vi "Find some Public API VI.vi"(7 "Theme":bool=TRUE, 8 "Public Api file index":i32, 9 "Library in":refnum<vi>, 10 "Target":refnum<vi>, 11 "App Ref":refnum<vi>) -> ()   [LabVIEW 2019, in "Panther Dashboard.lvlib"]
uses:
  Panther Dashboard.lvlib
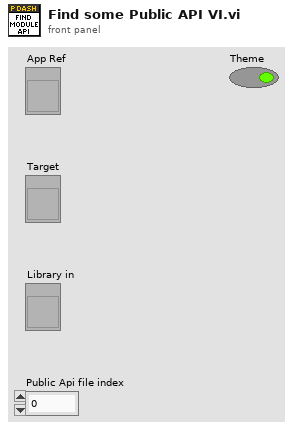
[diagram p1: front panel]
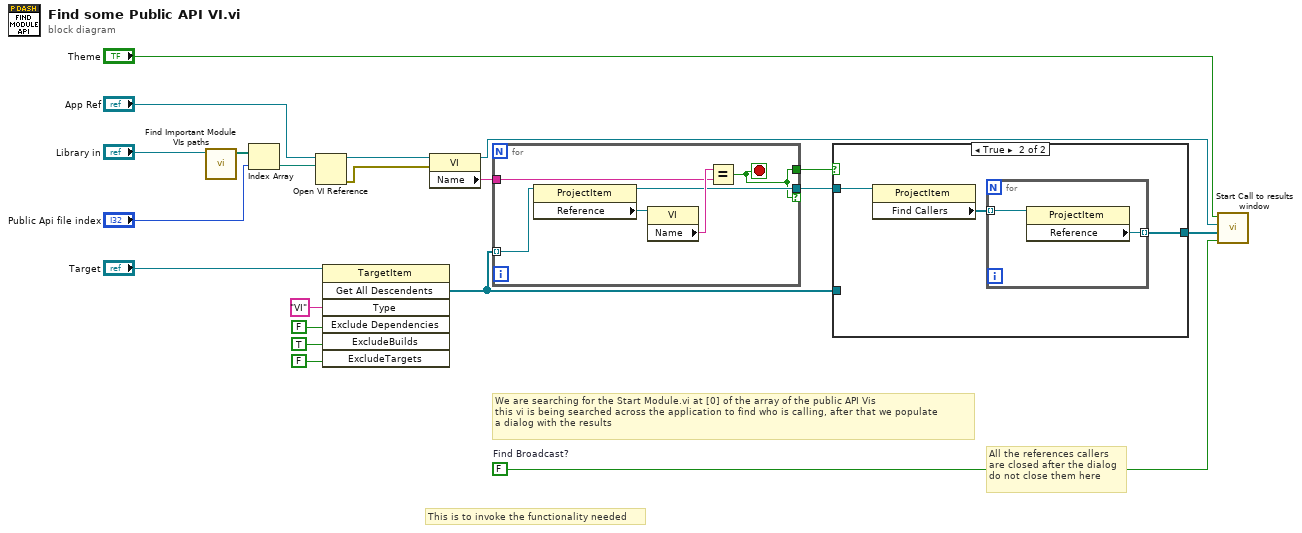
[diagram p0: block diagram]
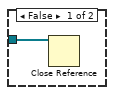
[diagram p2: hidden frame]
diagram:
  w4 = FALSE  # Find Broadcast?
  # "All the references callers\nare closed after the dialog\ndo not close them here"
  # "This is to invoke the functionality needed"
  # "We are searching for the Start Module.vi at [0] of the array of the public API Vis\nthis vi is being searched across the application to find who is calling, after that we populate\na dialog with the results"
  n1 = call "Find Important Module VIs paths.vi"("Library in"="Library in") -> ("Public API VIs Paths"=w18:path[])  [unwired: 10 in]
  n2 = Index Array(array=w18, index="Public Api file index") -> (element=w17:path)
  n3 = Open VI Reference(application reference (local)="App Ref", vi path=w17) -> (vi reference=w5:refnum<vi>, error out=w20:errorcluster)  [unwired: 4 in]
  n4 = invoke class="TargetItem" method="Get All Descendents"(reference="Target", "Type"="VI", "Exclude Dependencies"=FALSE ("ExcludeDependencies"), "ExcludeBuilds"=TRUE, "ExcludeTargets"=FALSE) -> ("All Descendents"=w6:refnum<vi>[])  [unwired: 2 in, 6 out]
  n5 = property class="VI"(reference=w5, error in=w20) -> (reference out=w1:refnum<vi>, "Name"=w13:string)  [unwired: 1 out]
  n6 = for {
    tunnel: w6 -> [w26] mode=indexing
    tunnel: w13 -> [w23]
    tunnel: [w22] -> w11 if=w21
    tunnel: [w21] -> w12
    stop <- w21 stop-if-true
    n7 = property class="ProjectItem"(reference=w26) -> (reference out=w22:refnum<vi>, "Reference"=w25:refnum<vi>)  [unwired: 1 in, 1 out]
    n8 = property class="VI"(reference=w25) -> ("Name"=w24:string)  [unwired: 1 in, 2 out]
    n9 = Equal?(x=w24, y=w23) -> (x = y?=w21:bool)
  }
  n10 = case shown="True" w12 {
    tunnel: w11 -> [_ w30]
    tunnel: w6 -> [w27 _]
    tunnel: [_ w28] -> w3
    frame False {
      n11 = Close Reference(reference=w27) -> ()  [unwired: 1 in, 1 out]
    }
    frame True {
      n12 = property class="ProjectItem"(reference=w30) -> ("Find Callers"=w29:refnum<vi>[])  [unwired: 1 in, 2 out]
      n13 = for {
        tunnel: w29 -> [w32] mode=indexing
        tunnel: [w31] -> w28 mode=indexing
        n14 = property class="ProjectItem"(reference=w32) -> ("Reference"=w31:refnum<vi>)  [unwired: 1 in, 2 out]
      }
    }
  }
  n15 = call "Start Call to results window.vi"("Find Broadcast?"=w4, "Request VI Callers"=w3, "Event"=w1, "Theme"="Theme") -> ()  [unwired: 8 in]
